vi "DoAttack.vi"(8 "error in (no error)":errorcluster, 10 "Rival":refnum<class "Peasant.lvclass">, 11 "Weapon in":refnum<class "Weapon.lvclass">) -> (0 "error out":errorcluster, 2 "Rival":refnum<class "Peasant.lvclass">, 3 "Weapon out":refnum<class "Weapon.lvclass">)   [LabVIEW 2021, in "Weapon.lvclass"]
uses:
  Weapon.lvclass
  Peasant/Peasant.lvclass
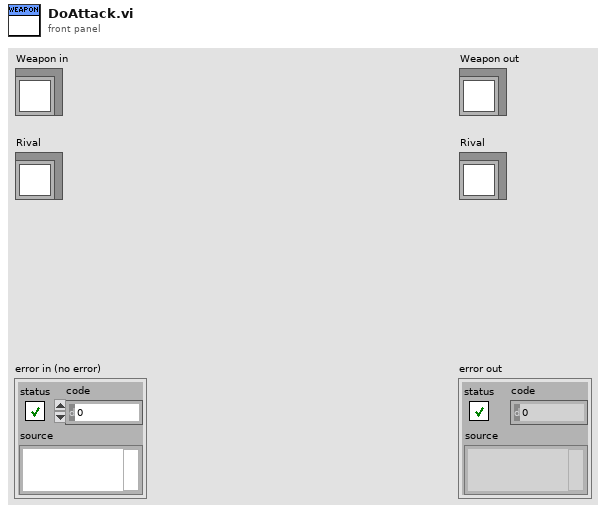
[diagram p1: front panel]
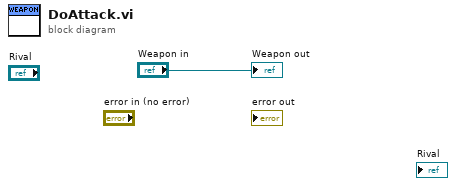
[diagram p0: block diagram]
diagram:
  "Weapon out" <- "Weapon in"
